vi "Update State Description.vi"(8 "error in (no error)":errorcluster, 9 "description":string, 10 "State":string, 11 "Channel Ref in":T1 format="%.0x") -> (0 "error out":errorcluster, 3 "Channel Ref out":T1=18446744073709551615 format="%.0x")   [LabVIEW 2017, in "SLSC Switch Scripting.lvlib"]
uses:
  SLSC Switch Scripting.lvlib
  <vilib>/NI Veristand/Custom Device API/Custom Device Item Ref.ctl
  <vilib>/NI VeriStand/Custom Device API/Custom Device API.lvlib
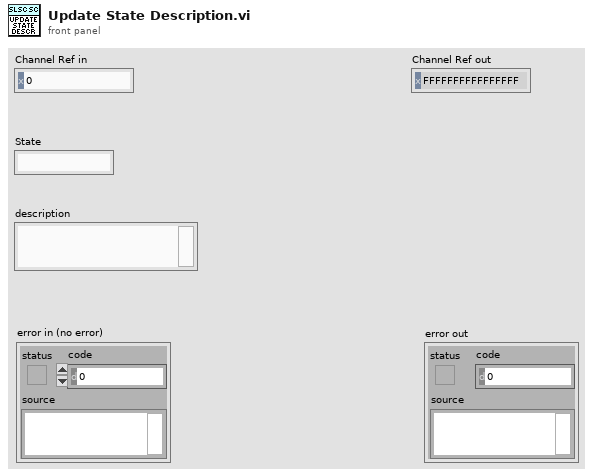
[diagram p1: front panel]
types:
  T1 = typedef "Custom Device API.lvlib/Custom Device Item Ref.ctl" = u64
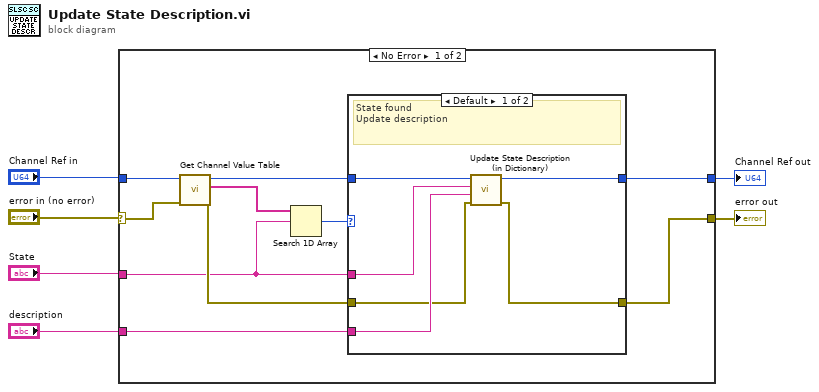
[diagram p0: block diagram]
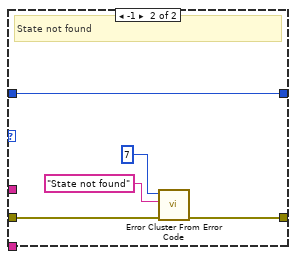
[diagram p2: hidden frame]
diagram:
  n1 = case shown="No Error" "error in (no error)" {
    selector: "error in (no error)" -> [w15 w29]
    tunnel: [w11 w29] -> w2
    tunnel: "Channel Ref in" -> [w16 w28]
    tunnel: [w12 w28] -> w1
    tunnel: "State" -> [w9 _]
    tunnel: "description" -> [w8 _]
    frame No Error {
      n2 = call "Get Channel Value Table.vi"("error in (no error)"=w15, "Channel Ref in"=w16) -> ("error out"=w13:errorcluster, "States"=w10:string[], "Channel Ref out"=w14:T1)  [unwired: 6 in, 1 out]
      n3 = Search 1D Array(1D array=w10, element=w9) -> (index of element=w7:i32)  [unwired: 1 in]
      n4 = case shown="Default" w7 {
        tunnel: w14 -> [w22 w23]
        tunnel: w13 -> [w18 w25]
        tunnel: [w21 w23] -> w12
        tunnel: [w17 w24] -> w11
        tunnel: w8 -> [w19 _]
        tunnel: w9 -> [w20 _]
        frame Default {
          # "State found\nUpdate description"
          n5 = call "Update State Description (in Dictionary).vi"("error in (no error)"=w18, "description"=w19, "State"=w20, "Channel Ref in"=w22) -> ("error out"=w17:errorcluster, "Channel Ref out"=w21:T1)  [unwired: 6 in]
        }
        frame -1 {
          # "State not found"
          n6 = call <vilib>:"Error Cluster From Error Code.vi"("error in (no error)"=w25, "error message (\"\")"="State not found" ("error message (\"\")"), "error code (0)"=7) -> ("error out"=w24:errorcluster)  [unwired: 6 in]
        }
      }
    }
    frame Error {
    }
  }
  "Channel Ref out" <- w1
  "error out" <- w2
